vi "Ch_data_title_pattern 16 (SubVI).vi"(9 "Единица измерений":string) -> (0 "error out":errorcluster, 2 "Path":path, 3 "Byte Stream File out":refnum<file>)   [LabVIEW 8.6]
panel:
  in  "error in":errorcluster
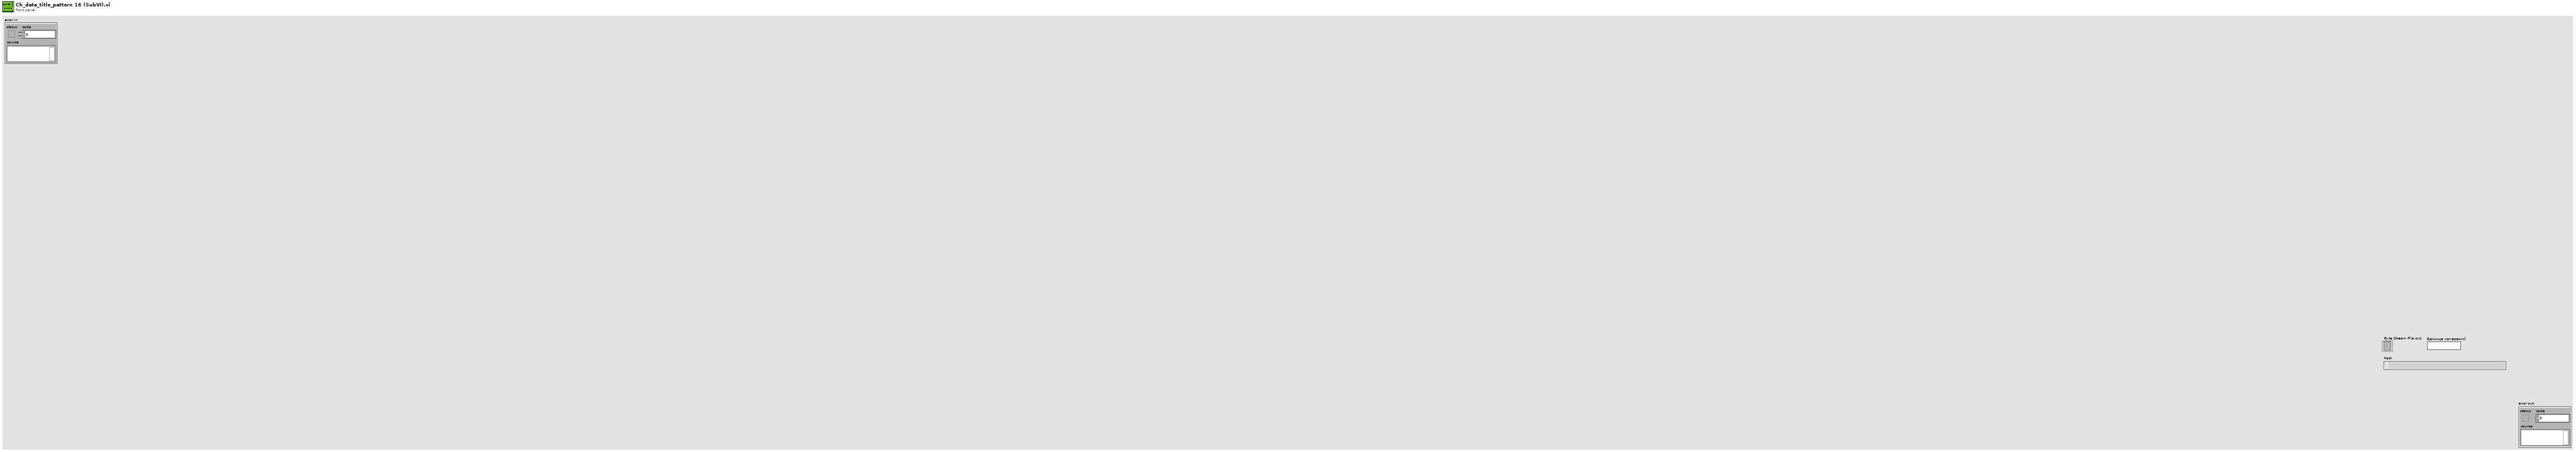
[diagram p1: front panel]
types:
  T1 = enum16{"open", "replace", "create", "open or create", "replace or create", "replace or create with confirmation"}
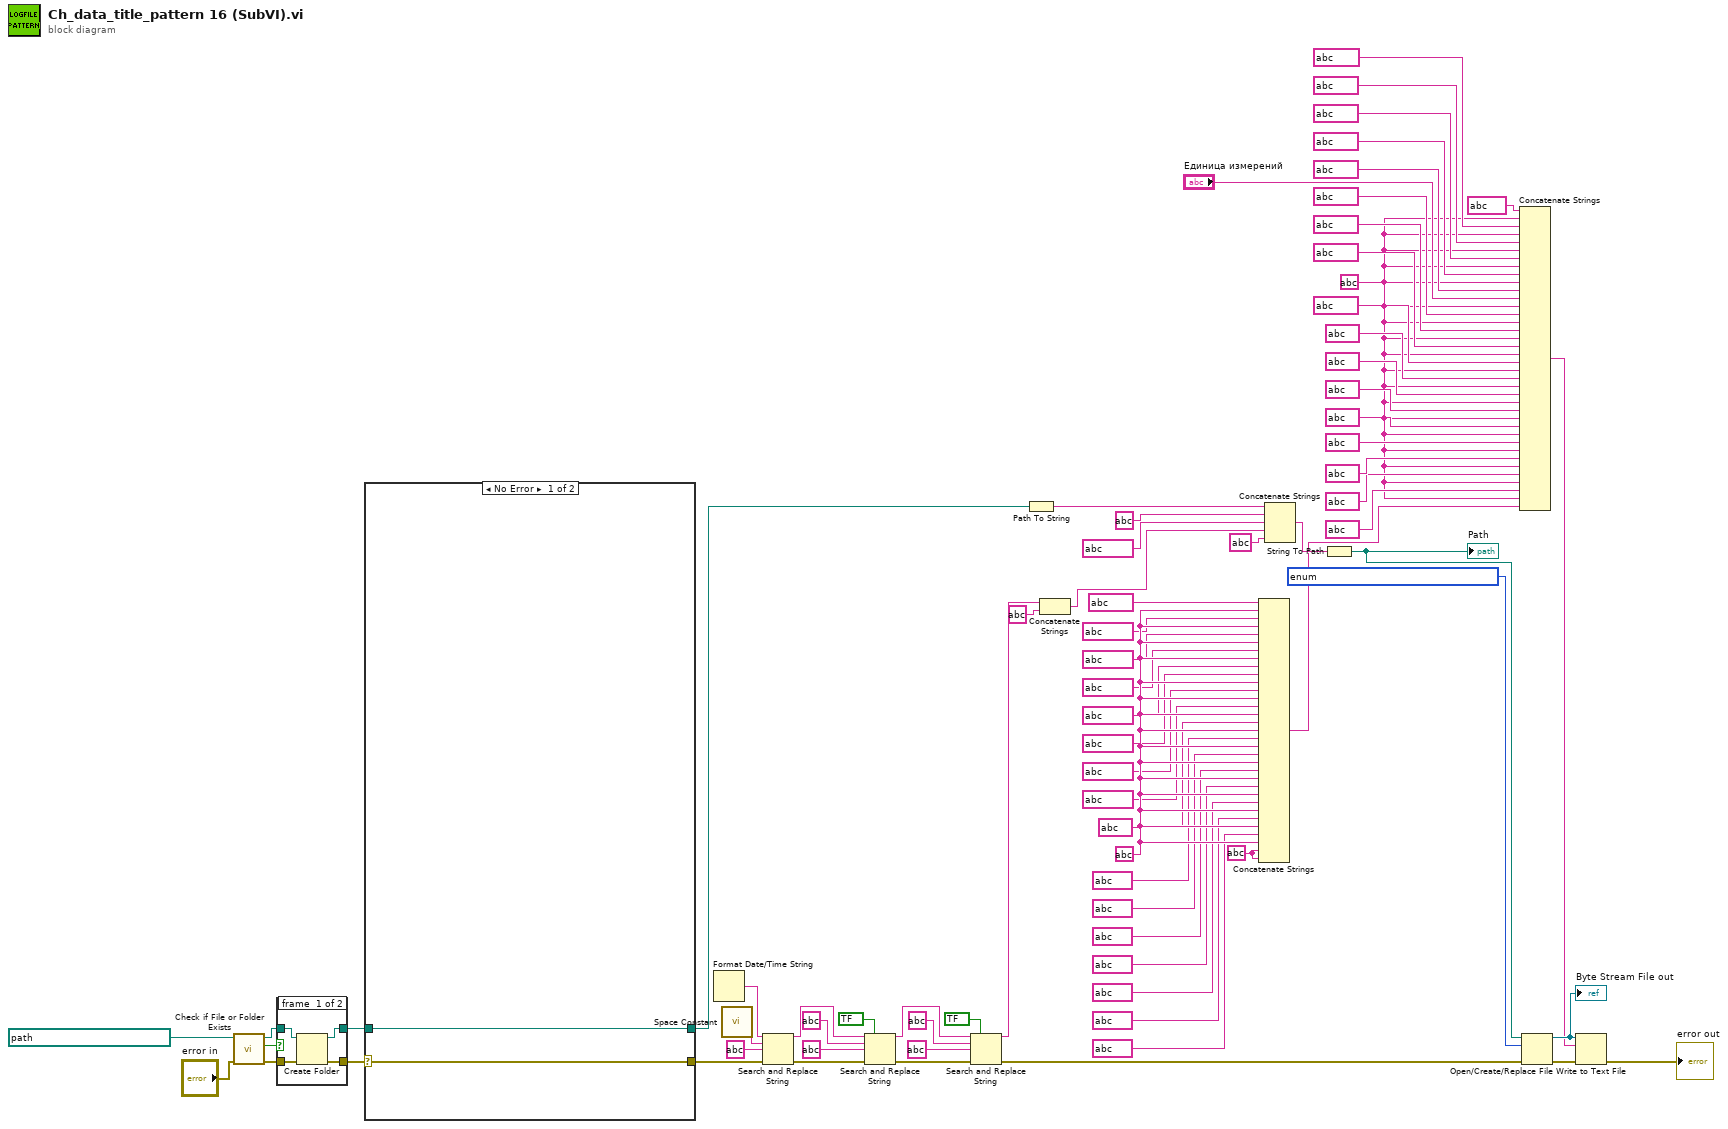
[diagram p0: block diagram]
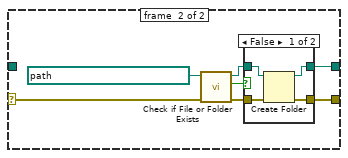
[diagram p2: hidden frame]
diagram:
  w19 = string ?
  w20 = string ?
  w2 = string ?
  n1 = call <vilib>:"Check if File or Folder Exists.vi"("error in (no error)"="error in", "path"=path ? ("path (use dialog)")) -> ("error out"=w63:errorcluster, "file or folder exists?"=w61:bool, "dup path"=w64:path)  [unwired: 7 out]
  n2 = case shown="True" w61 {
    tunnel: [w80 w82] -> w59
    tunnel: w64 -> [w79 w82]
    tunnel: w63 -> [w78 w81]
    tunnel: [w77 w81] -> w60
    frame #0 {
      n3 = Create Folder(path (use dialog)=w79, error in=w78) -> (created path=w80:path, error out=w77:errorcluster)  [unwired: 2 out]
    }
    frame #1 {
    }
  }
  n4 = case shown="No Error" w60 {
    selector: w60 -> [w83 w85]
    tunnel: w59 -> [w84 _]
    tunnel: [w84 w88] -> w35
    tunnel: [w83 w87] -> w36
    frame #0 {
    }
    frame #1 {
      n5 = call <vilib>:"Check if File or Folder Exists.vi"("error in (no error)"=w85, "path"=path ? ("path (use dialog)")) -> ("error out"=w90:errorcluster, "file or folder exists?"=w89:bool, "dup path"=w91:path)  [unwired: 7 out]
      n6 = case shown="False" w89 {
        tunnel: [w95 w97] -> w88
        tunnel: w91 -> [w94 w97]
        tunnel: w90 -> [w93 w96]
        tunnel: [w92 w96] -> w87
        frame #0 {
          n7 = Create Folder(path (use dialog)=w94, error in=w93) -> (created path=w95:path, error out=w92:errorcluster)  [unwired: 2 out]
        }
        frame #1 {
        }
      }
    }
  }
  n8 = Format Date/Time String() -> (date/time string=w57:string)  [unwired: 3 out]
  n9 = call <vilib>:"Space Constant.vi"() -> ("String"=w38:string)
  n10 = Search and Replace String(input string=w57, search string=w38, replace string=string ? ("replace string (\"\")"), error in=w36) -> (result string=w40:string, error out=w50:errorcluster)  [unwired: 6 out]
  n11 = Search and Replace String(replace all?=bool ? ("replace all? (F)"), input string=w40, search string=string ?, replace string=string ? ("replace string (\"\")"), error in=w50) -> (result string=w47:string, error out=w51:errorcluster)  [unwired: 5 out]
  n12 = Search and Replace String(replace all?=bool ? ("replace all? (F)"), input string=w47, search string=string ?, replace string=string ? ("replace string (\"\")"), error in=w51) -> (result string=w52:string, error out=w34:errorcluster)  [unwired: 5 out]
  n13 = Path To String(path=w35) -> (string=w48:string)
  n14 = Concatenate Strings(w52, string ? ("string")) -> (w55:string)
  n15 = Concatenate Strings(string ? ("string"), w19, string ? ("string"), w19, string ? ("string"), w19, string ? ("string"), w19, string ? ("string"), string ? ("string"), w19, string ? ("string"), w19, string ? ("string"), w19, string ? ("string"), w19, string ? ("string"), w19, string ? ("string"), w19, string ? ("string"), w19, string ? ("string"), w19, string ? ("string"), w19, string ? ("string"), w19, string ? ("string"), w19, w2, w2) -> (w1:string)
  n16 = Concatenate Strings(w48, string ? ("string"), string ? ("string"), w55, string ? ("default name")) -> (w37:string)
  n17 = String To Path(string=w37) -> (path=w33:path)
  "Path" <- w33
  n18 = Concatenate Strings(string ? ("string"), w20, string ? ("string"), w20, string ? ("string"), w20, string ? ("string"), w20, string ? ("string"), w20, string ? ("string"), "Единица измерений", w20, string ? ("string"), w20, string ? ("string"), w20, string ? ("string"), w20, string ? ("string"), w20, string ? ("string"), w20, string ? ("string"), w20, string ? ("string"), w20, string ? ("string"), w20, string ? ("string"), w20, string ? ("string"), w20, string ? ("string"), w20, string ? ("string"), w20, w1) -> (w67:string)
  n19 = Open/Create/Replace File(file path (use dialog)=w33, error in=w34, operation (0:open)=T1 ?) -> (refnum out=w70:refnum<file>, error out=w68:errorcluster)  [unwired: 4 out]
  "Byte Stream File out" <- w70
  n20 = Write to Text File(file (use dialog)=w70, text=w67, error in=w68) -> (error out=→"error out":errorcluster)  [unwired: 3 out]
